vi "Get SMO HELP getAll.vi"(8 "error in (no error)":errorcluster, 11 "Instrument in":refnum<class "Instrument.lvclass">) -> (0 "error out":errorcluster, 2 "response cluster":variant, 3 "Instrument out":refnum<class "Instrument.lvclass">)   [LabVIEW 2019, in "Instrument.lvlib" / "Instrument.lvclass"]
uses:
  Instrument.lvclass
  <vilib>/ciozi137/JSON-Schema/JSON-Schema.lvlib
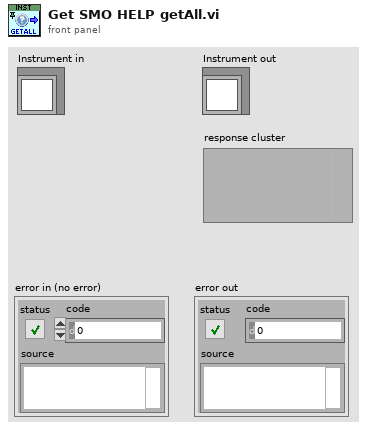
[diagram p1: front panel]
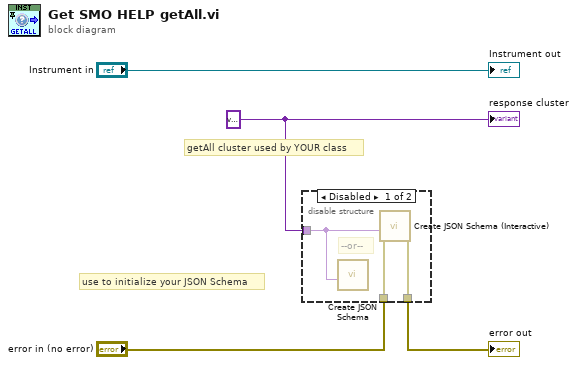
[diagram p0: block diagram]
diagram:
  w3 = variant
  # "use to initialize your JSON Schema"
  # "getAll cluster used by YOUR class"
  n1 = disable-structure shown="Disabled" {
    disable-tunnel: w3 -> [w5 _]
    disable-tunnel: "error in (no error)" -> [w7 _]
    disable-tunnel: [w6 _] -> w1
    frame Disabled {
      # "--or--"
      n2 = call <vilib>:"Create JSON Schema.vi"("LV Object"=w5) -> ()  [unwired: 10 in, 1 out]
      n3 = call <vilib>:"Create JSON Schema (Interactive).vi"("error in (no error)"=w7, "LV Object"=w5) -> ("error out"=w6:errorcluster)  [unwired: 8 in, 1 out]
    }
    frame Enabled {
    }
  }
  "error out" <- w1
  "Instrument out" <- "Instrument in"
  "response cluster" <- w3
